vi "注册用户.vi"() -> ()   [LabVIEW 2019]
panel:
  out "Data":string[][](array[string])
  out "error out":errorcluster
  in  "返回":bool
  in  "注册":bool
  in  "确认密码":string
  in  "密       码":string
  in  "用 户 名":string
  # "用户注册"
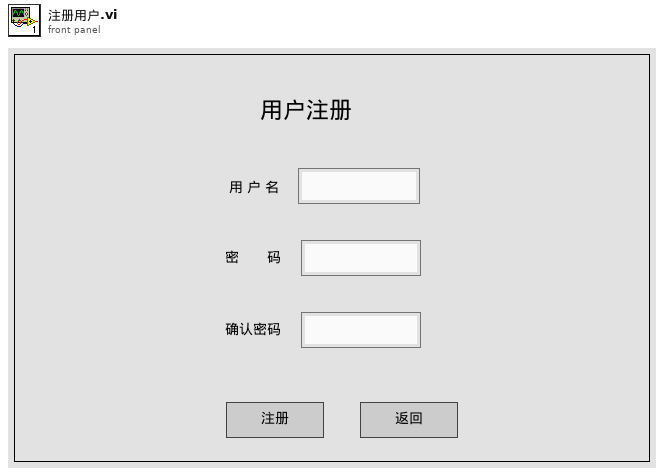
[diagram p1: front panel]
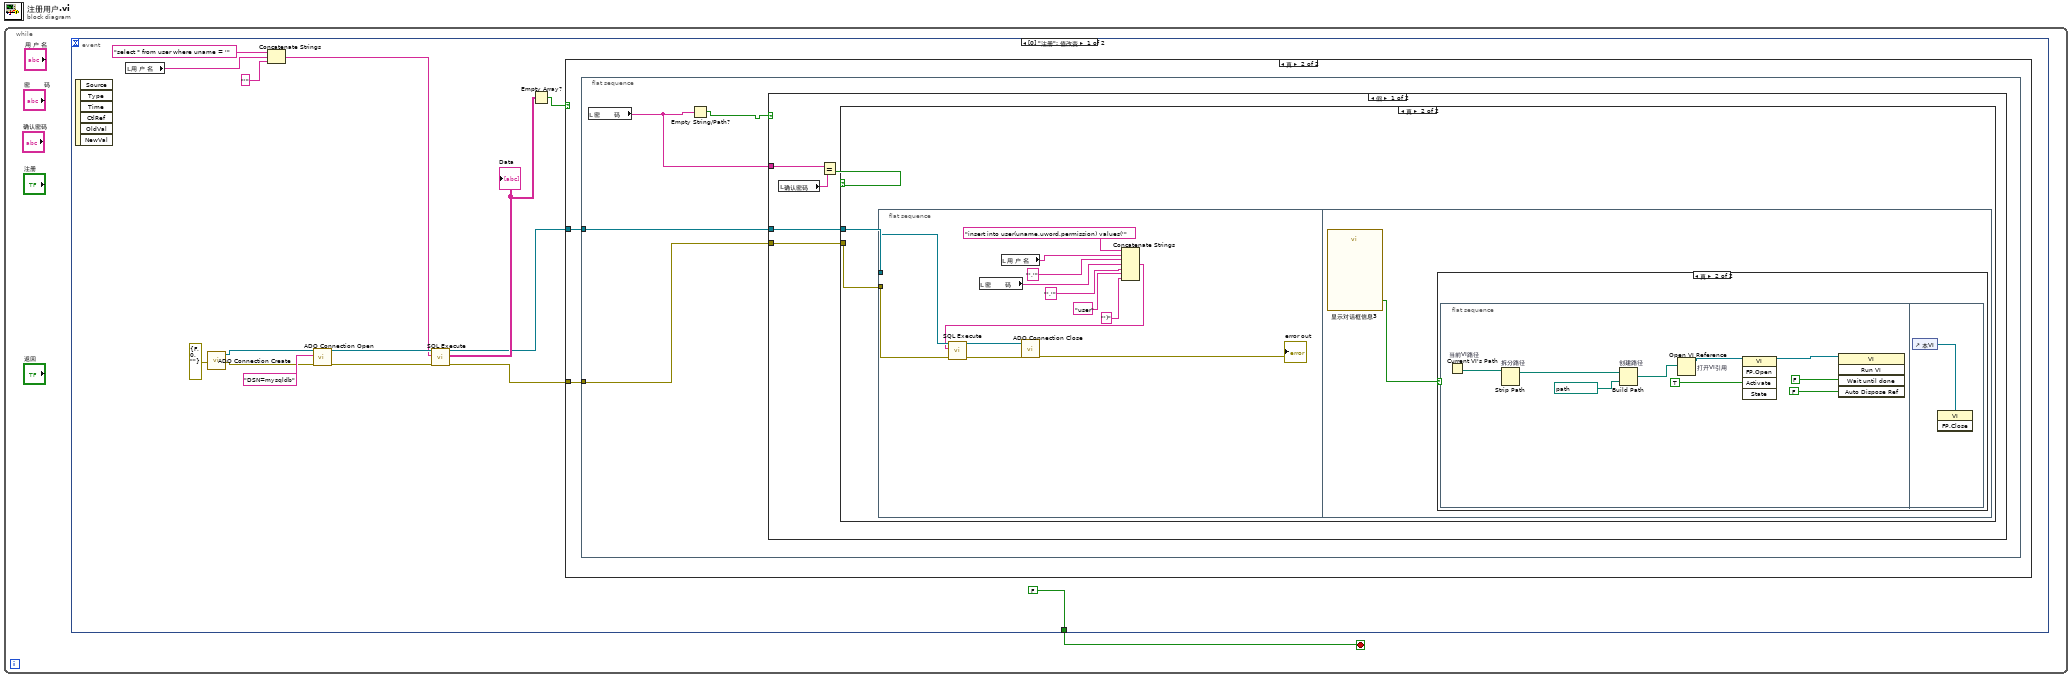
[diagram p0: block diagram]
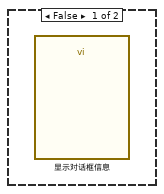
[diagram p2: hidden frame]
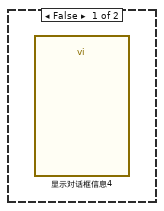
[diagram p3: hidden frame]
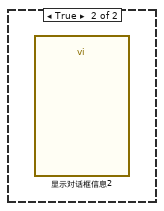
[diagram p5: hidden frame]
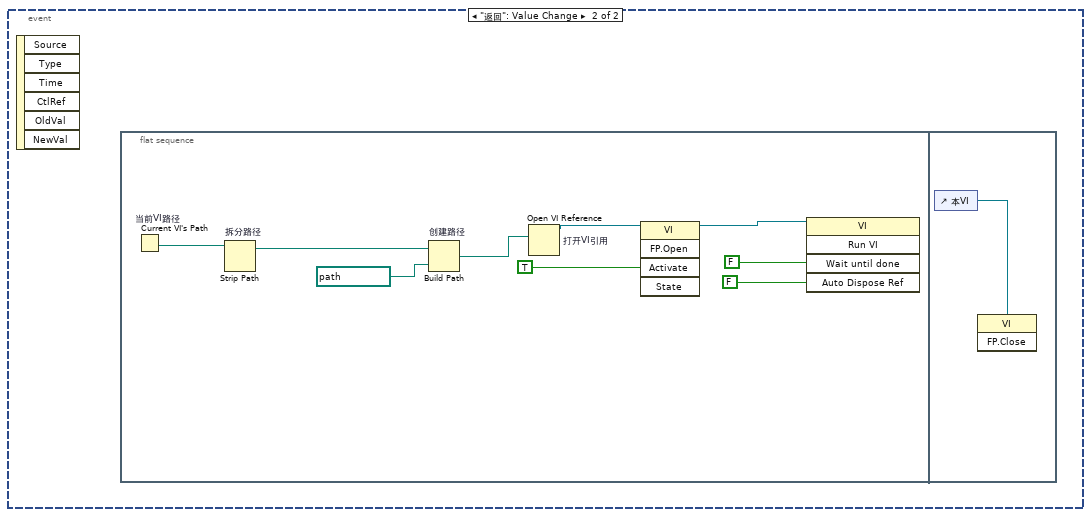
[diagram p6: hidden frame]
diagram:
  n1 = while {
    stop <- w1 stop-if-true
    n2 = event shown="[0] \"注册\": 值改变" {
      selector: _ -> [_ _]
      dyn-events: _ -> [_ _]
      timeout: _ -> [_ _]
      tunnel: [FALSE _] -> w1
      event "注册": Value Change {
        n3 = event-data() -> ()  [unwired: 1 in, 6 out]
        n4 = local read "用 户 名"() -> (w10:string)
        n5 = call <userlib>:"ADO Connection Create.vi"("error in (no error)"=errorcluster {"status"=FALSE, "code"=0, "source"=""}) -> ("error out"=w13:errorcluster, "ADODB._Connection Out"=w16:refnum<k7>)  [unwired: 9 in]
        n6 = Concatenate Strings("select * from user where uname = '", w10, "'" ("字符串")) -> (w8:string)
        n7 = call <userlib>:"ADO Connection Open.vi"("error in (no error)"=w13, "ConnectionString"="DSN=mysqldb", "ADODB._Connection In"=w16) -> ("error out"=w12:errorcluster, "ADODB._Connection Out"=w15:refnum<k7>)  [unwired: 7 in]
        n8 = call <userlib>:"SQL Execute.vi"("error in (no error)"=w12, "Command Text"=w8, "ADODB._Connection In"=w15) -> ("error out"=w3:errorcluster, "Data"=w6:string[][], "ADODB._Connection Out"=w2:refnum<k7>)  [unwired: 5 in, 1 out]
        "Data" <- w6
        n9 = Empty Array?(array=w6) -> (empty?=w5:bool)
        n10 = case shown="真" w5 {
          tunnel: w3 -> [_ w18]
          tunnel: w2 -> [_ w17]
          frame False {
            n11 = call "显示对话框信息"() -> ()  [unwired: 10 in, 2 out]
          }
          frame True {
            n12 = flat-sequence {
              tunnel: w18 -> [w20]
              tunnel: w17 -> [w19]
              frame #0 {
                n13 = local read "密       码"() -> (w21:string)
                n14 = Empty String/Path?(string/path=w21) -> (empty?=w22:bool)
                n15 = case shown="假" w22 {
                  tunnel: w21 -> [w26 _]
                  tunnel: w20 -> [w24 _]
                  tunnel: w19 -> [w23 _]
                  frame False {
                    n16 = local read "确认密码"() -> (w27:string)
                    n17 = Equal?(x=w26, y=w27) -> (x = y?=w25:bool)
                    n18 = case shown="真" w25 {
                      tunnel: w24 -> [_ w29]
                      tunnel: w23 -> [_ w28]
                      frame False {
                        n19 = call "显示对话框信息4"() -> ()  [unwired: 10 in, 2 out]
                      }
                      frame True {
                        n20 = flat-sequence {
                          tunnel: w29 -> [w40]
                          tunnel: w28 -> [w39]
                          frame #0 {
                            n21 = local read "密       码"() -> (w36:string)
                            n22 = local read "用 户 名"() -> (w38:string)
                            n23 = Concatenate Strings("insert into user(uname,uword,permission) values('", w38, "','" ("字符串"), w36, "','" ("字符串"), "user", "')" ("字符串")) -> (w34:string)
                            n24 = call <userlib>:"SQL Execute.vi"("error in (no error)"=w40, "Command Text"=w34, "ADODB._Connection In"=w39) -> ("error out"=w42:errorcluster, "ADODB._Connection Out"=w41:refnum<k7>)  [unwired: 5 in, 2 out]
                            n25 = call <userlib>:"ADO Connection Close.vi"("error in (no error)"=w42, "ADODB._Connection In"=w41) -> ("error out"=→"error out":errorcluster)  [unwired: 8 in, 1 out]
                          }
                          frame #1 {
                            n26 = call "显示对话框信息3"() -> ("确定"=w43:bool)  [unwired: 10 in, 1 out]
                            n27 = case shown="真" w43 {
                              frame False {
                              }
                              frame True {
                                n28 = flat-sequence {
                                frame #0 {
                                n29 = Current VI's Path "当前VI路径"() -> (path=w45:path)
                                n30 = Strip Path "拆分路径"(path=w45) -> (stripped path=w44:path)  [unwired: 1 out]
                                n31 = Build Path "创建路径"(base path=w44, name or relative path=path "用户登录.vi") -> (appended path=w47:path)
                                n32 = Open VI Reference "打开VI引用"(vi path=w47) -> (vi reference=w46:refnum<vi>)  [unwired: 5 in, 1 out]
                                n33 = invoke class="VI" method="FP.Open"(reference=w46, "Activate"=TRUE) -> (reference out=w50:refnum<vi>)  [unwired: 3 in, 4 out]
                                n34 = invoke class="VI" method="Run VI"(reference=w50, "Wait until done"=FALSE, "Auto Dispose Ref"=FALSE) -> ()  [unwired: 2 in, 5 out]
                                }
                                frame #1 {
                                n35 = control-ref of="本VI"() -> (w53:refnum<vi>)
                                n36 = invoke class="VI" method="FP.Close"(reference=w53) -> ()  [unwired: 2 in, 3 out]
                                }
                                }
                              }
                            }
                          }
                        }
                      }
                    }
                  }
                  frame True {
                    n37 = call "显示对话框信息2"() -> ()  [unwired: 10 in, 2 out]
                  }
                }
              }
            }
          }
        }
      }
      event "返回": Value Change {
        n38 = event-data() -> ()  [unwired: 1 in, 6 out]
        n39 = flat-sequence {
          frame #0 {
            n40 = Current VI's Path "当前VI路径"() -> (path=w55:path)
            n41 = Strip Path "拆分路径"(path=w55) -> (stripped path=w54:path)  [unwired: 1 out]
            n42 = Build Path "创建路径"(base path=w54, name or relative path=path "用户登录.vi") -> (appended path=w57:path)
            n43 = Open VI Reference "打开VI引用"(vi path=w57) -> (vi reference=w56:refnum<vi>)  [unwired: 5 in, 1 out]
            n44 = invoke class="VI" method="FP.Open"(reference=w56, "Activate"=TRUE) -> (reference out=w60:refnum<vi>)  [unwired: 3 in, 4 out]
            n45 = invoke class="VI" method="Run VI"(reference=w60, "Wait until done"=FALSE, "Auto Dispose Ref"=FALSE) -> ()  [unwired: 2 in, 5 out]
          }
          frame #1 {
            n46 = control-ref of="本VI"() -> (w63:refnum<vi>)
            n47 = invoke class="VI" method="FP.Close"(reference=w63) -> ()  [unwired: 2 in, 3 out]
          }
        }
      }
    }
  }
